vi "IntakeExecute.vi"() -> ()   [LabVIEW 2023]
uses:
  <vilib>/Rock Robotics/WPI/ThirdParty/REV Robotics/REVLib/Typedef/Spark MAX Control Type.ctl
panel:
  in  "error in (no error)":errorcluster
  out "error out":errorcluster
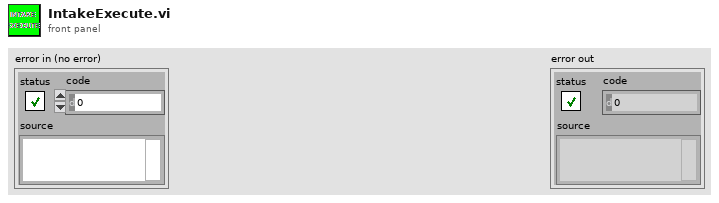
[diagram p1: front panel]
types:
  T1 = typedef "Spark MAX Control Type.ctl" = enum16{"Percent VBus", "Voltage", "Velocity", "Position", "Smart Motion", "Current", "Smart Velocity", "MAXMotion Position", "MAXMotion Velocity"}
  T2 = typedef "WPI_MotorControlDeviceRef.ctl" = cluster{"DeviceStatus":errorcluster, "Type":T3, "PWM":cluster{"PWM Channel":T4, "DeadBand":T5}, "CAN":cluster{"Device Number":u8, "SetOutput VI Ref":variant, "GetOutput VI Ref":variant, "Enable VI Ref":variant, "Disable VI Ref":variant, "Data":variant}, "Invert":bool, "DIO PWM":cluster{"PWM \"Enable\" Channel":T4, "DIOChannel":T6, "PWM Rate":dbl}}
  T3 = typedef "WPI_MotorControlType.ctl" = enum16{"PWM", "CAN", "DIO PWM"}
  T4 = typedef "FPGA_DIOPWMChannel.ctl" = enum8{"PWM 0", "PWM 1", "PWM 2", "PWM 3", "PWM 4", "PWM 5", "PWM 6", "PWM 7", "PWM 8", "PWM 9", "PWM MXP 0", "PWM MXP 1", "PWM MXP 2", "PWM MXP 3", "PWM MXP 4", "PWM MXP 5", "PWM MXP 6", "PWM MXP 7", "PWM MXP 8", "PWM MXP 9", "Invalid"}
  T5 = typedef "WPI_PWMDeadband.ctl" = cluster{"Name":string, "maxPositivePwm":i32, "minPositivePwm":i32, "centerPwm":i32, "maxNegativePwm":i32, "minNegativePwm":i32, "angularRange":u16}
  T6 = typedef "FPGA_DIOChannel.ctl" = enum8{"DIO 0", "DIO 1", "DIO 2", "DIO 3", "DIO 4", "DIO 5", "DIO 6", "DIO 7", "DIO 8", "DIO 9", "DIO MXP 0", "DIO MXP 1", "DIO MXP 2", "DIO MXP 3", "DIO MXP 4", "DIO MXP 5", "DIO MXP 6", "DIO MXP 7", "DIO MXP 8", "DIO MXP 9", "DIO MXP 10", "DIO MXP 11", "DIO MXP 12", "DIO MXP 13", "DIO MXP 14", "DIO MXP 15", "SPI Port CS1", "SPI Port CS2", "SPI Port CS3", "SPI Port MISO", "SPI Port MOSI", "Invalid"}
  T7 = typedef "WPI_SwitchDevRef.ctl" = cluster{"DevStatus":errorcluster, "DIO Channel":T6, "CntIndex":T8, "Normally Closed":bool}
  T8 = typedef "FPGA_CounterCtrSystemIndex.ctl" = enum8{"Ctr 0", "Ctr 1", "Ctr 2", "Ctr 3", "Ctr 4", "Ctr 5", "Ctr 6", "Ctr 7", "Invalid"}
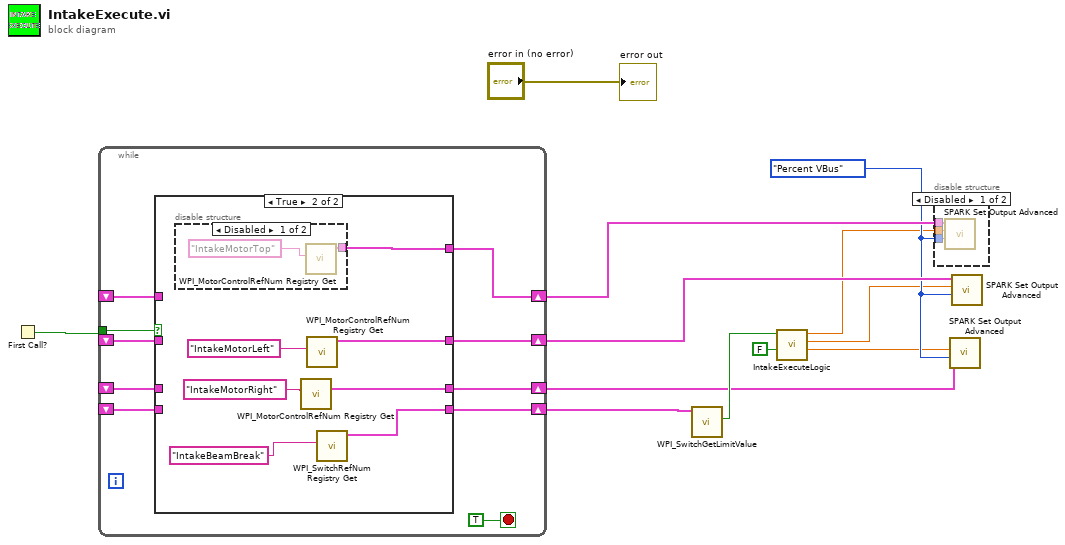
[diagram p0: block diagram]
diagram:
  w5 = Spark_MAX_Control_Type."Percent VBus" ("Control Mode")
  n1 = First Call?() -> (First Call?: T/F=w11:bool)
  n2 = while {
    tunnel: w11 -> [w21]
    shift-right: [w22] -> w7
    shift-left: _ -> [w20]
    shift-right: [w18] -> w8
    shift-left: _ -> [w17]
    shift-right: [w16] -> w6
    shift-left: _ -> [w15]
    shift-right: [w14] -> w10
    shift-left: _ -> [w13]
    stop <- TRUE stop-if-true
    n3 = case shown="True" w21 {
      tunnel: [w26 w31] -> w22
      tunnel: w20 -> [w26 _]
      tunnel: [w25 w30] -> w18
      tunnel: w17 -> [w25 _]
      tunnel: [w24 w29] -> w16
      tunnel: w15 -> [w24 _]
      tunnel: [w23 w27] -> w14
      tunnel: w13 -> [w23 _]
      frame False {
      }
      frame True {
        n4 = disable-structure shown="Disabled" {
          disable-tunnel: [w34 _] -> w29
          frame Disabled {
            n5 = call <vilib>:"WPI_MotorControlRefNum Registry Get.vi"("refnum name"="IntakeMotorTop") -> ("MotorControlDevRef"=w34:T2)  [unwired: 9 in, 1 out]
          }
          frame Enabled {
          }
        }
        n6 = call <vilib>:"WPI_MotorControlRefNum Registry Get.vi"("refnum name"="IntakeMotorRight") -> ("MotorControlDevRef"=w31:T2)  [unwired: 9 in, 1 out]
        n7 = call <vilib>:"WPI_MotorControlRefNum Registry Get.vi"("refnum name"="IntakeMotorLeft") -> ("MotorControlDevRef"=w30:T2)  [unwired: 9 in, 1 out]
        n8 = call <vilib>:"WPI_SwitchRefNum Registry Get.vi"("refnum name"="IntakeBeamBreak") -> ("SwitchDevRef"=w27:T7)  [unwired: 9 in, 1 out]
      }
    }
  }
  n9 = call <vilib>:"WPI_SwitchGetLimitValue.vi"("SwitchDevRef"=w10) -> ("Switch Pressed"=w9:bool)  [unwired: 8 in, 2 out]
  n10 = call "IntakeExecuteLogic.vi"("HaveAlgaeSensor"=FALSE ("HaveAlgae"), "HaveCoralSensor"=w9) -> ("MotorDemandRight"=w3:dbl, "MotorDemandLeft"=w4:dbl, "MotorDemandTop"=w2:dbl)  [unwired: 6 in, 1 out]
  n11 = disable-structure shown="Disabled" {
    disable-tunnel: w6 -> [w38 _]
    disable-tunnel: w5 -> [w37 _]
    disable-tunnel: w2 -> [w36 _]
    frame Disabled {
      n12 = call <vilib>:"SPARK Set Output Advanced.vi"("Control Mode"=w37, "Setpoint"=w36, "MotorControlDevRef"=w38) -> ()  [unwired: 7 in, 2 out]
    }
    frame Enabled {
    }
  }
  n13 = call <vilib>:"SPARK Set Output Advanced.vi"("Control Mode"=w5, "Setpoint"=w3, "MotorControlDevRef"=w7) -> ()  [unwired: 7 in, 2 out]
  n14 = call <vilib>:"SPARK Set Output Advanced.vi"("Control Mode"=w5, "Setpoint"=w4, "MotorControlDevRef"=w8) -> ()  [unwired: 7 in, 2 out]
  "error out" <- "error in (no error)"
